vi "Test Get Default Plugins.vi"(8 "error in (no error)":errorcluster, 11 "Configuration Manager Test in":refnum<class "Configuration Manager Test.lvclass">) -> (0 "error out":errorcluster, 3 "Configuration Manager Test out":refnum<class "Configuration Manager Test.lvclass">)   [LabVIEW 2020, in "Configuration Manager Test.lvclass"]
uses:
  Configuration Manager Test.lvclass
  C:/Program Files (x86)/National Instruments/LabVIEW 2020/vi.lib/Astemes/LUnit/Core/LUnit Test Case/Test Case.lvclass
  <vilib>/Astemes/LUnit/Core/LUnit Test Case/Test Case.lvclass/Test Case.ctl
  b78b68b9-28ec-4fcb-9b61-f705c7f0904e.vi
  <vilib>/Astemes/LUnit/Core/LUnit Test Case/Private/Append Pass Result.vi
  <vilib>/Astemes/LUnit/Core/LUnit Test Case/Private/Append Fail Result.vi
  b78b68b9-28ec-4fcb-9b61-f705c7f0904e.vi/9c5d11cd-9439-4240-a1ee-d9baace9c924.vi
  <vilib>/Astemes/LUnit/Core/LUnit Test Case/Private/Run In UI.vi
  <vilib>/Utility/error.llb/Clear Errors.vi
  source/User Interface/Configuration Manager/Configuration Manager.lvclass
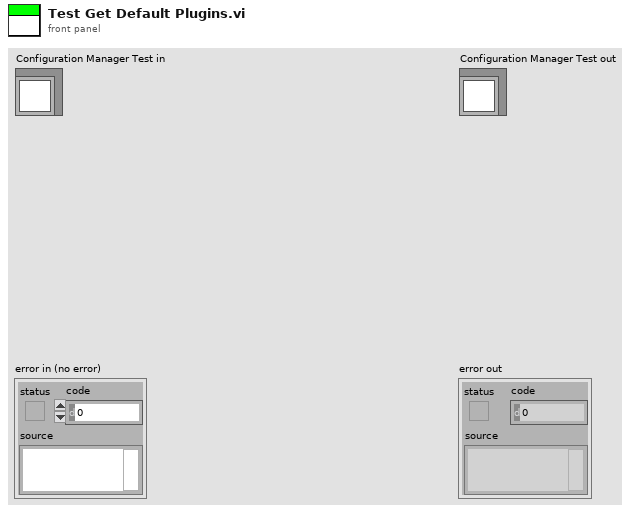
[diagram p1: front panel]
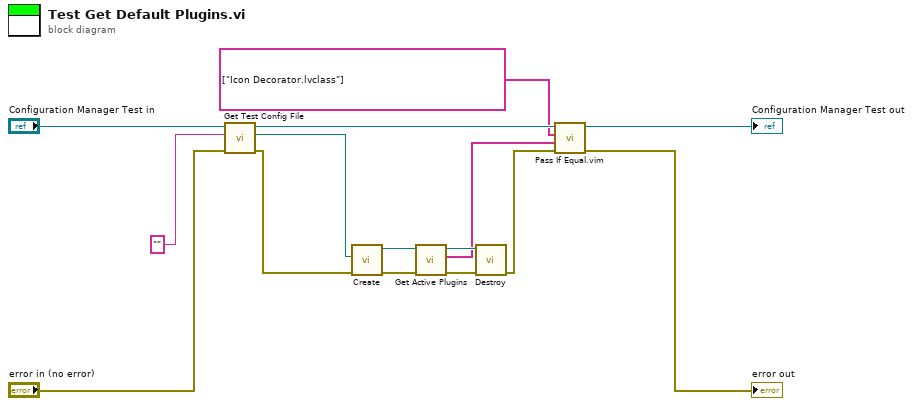
[diagram p0: block diagram]
diagram:
  n1 = call "Get Test Config File.vi"("error in (no error)"="error in (no error)", "File Content"="", "Configuration Manager Test in"="Configuration Manager Test in") -> ("error out"=w8:errorcluster, "File Path"=w3:path, "Configuration Manager Test out"=w5:refnum<class "Configuration Manager Test.lvclass">)  [unwired: 6 in]
  n2 = call "Create.vi"("error in (no error)"=w8, "configuration file path"=w3) -> ("error out"=w11:errorcluster, "Configuration Manager out"=w12:refnum<class "Configuration Manager.lvclass">)  [unwired: 8 in]
  n3 = call "Get Active Plugins.vi"("error in (no error)"=w11, "Configuration Manager In"=w12) -> ("error out"=w9:errorcluster, "Plugins"=w2:string[], "Configuration Manager Out"=w10:refnum<class "Configuration Manager.lvclass">)  [unwired: 7 in]
  n4 = call "Destroy.vi"("error in (no error)"=w9, "Configuration Manager In"=w10) -> ("error out"=w7:errorcluster)  [unwired: 9 in]
  n5 = call "Pass If Equal.vim"("error in (no error)"=w7, "Actual"=w2, "Expected"=string[] ["Icon Decorator.lvclass"], "LUnit Test Case In"=w5) -> ("error out"=→"error out":errorcluster, "LUnit Test Case Out"=→"Configuration Manager Test out":refnum<class "Configuration Manager Test.lvclass">)  [unwired: 6 in]
